vi "2022 Set Arm PID Constants.vi"(1 "error in (no error)":errorcluster, 2 "localConstantSpreadSheet":string[][](array[string]), 3 "robotID":string) -> (0 "error out":errorcluster)   [LabVIEW 2020]
uses:
  2023 Robot Global Data.vi
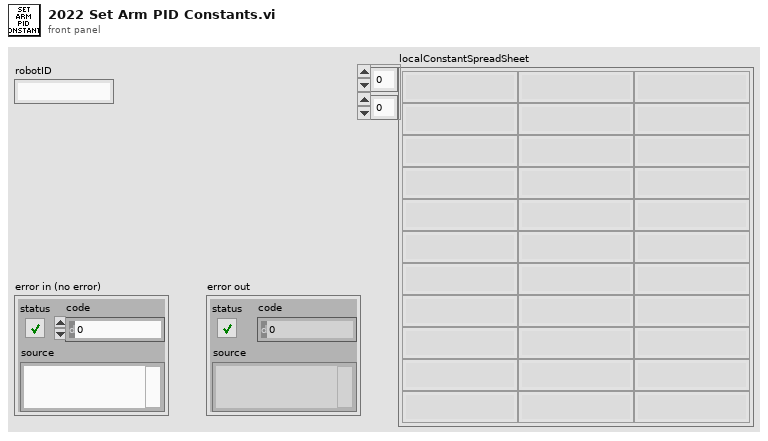
[diagram p1: front panel]
types:
  T1 = cluster{"P Gain":dbl, "I Gain":dbl, "D Gain":dbl, "F Gain":dbl, "I Zone":dbl, "Min Output":dbl, "Max Output":dbl}
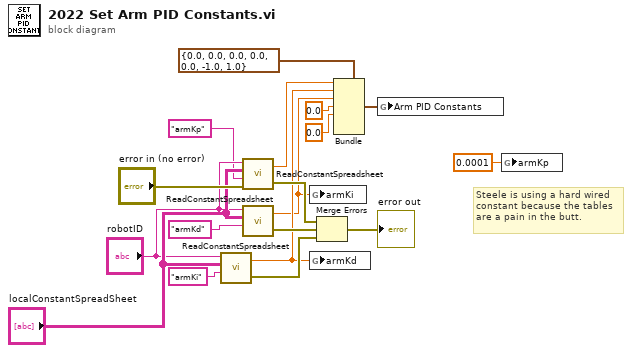
[diagram p0: block diagram]
diagram:
  # "Steele is using a hard wired\nconstant because the tables\nare a pain in the butt."
  n1 = call "ReadConstantSpreadsheet.vi"("Constant"="armKi", "2023ConstantSpreadSheet"="localConstantSpreadSheet", "Robot ID"="robotID") -> ("error out"=w16:errorcluster, "Constant Value"=w13:dbl)  [unwired: 1 in]
  n2 = call "ReadConstantSpreadsheet.vi"("error in"="error in (no error)", "Constant"="armKp", "2023ConstantSpreadSheet"="localConstantSpreadSheet", "Robot ID"="robotID") -> ("error out"=w14:errorcluster, "Constant Value"=w2:dbl)
  n3 = call "ReadConstantSpreadsheet.vi"("Constant"="armKd", "2023ConstantSpreadSheet"="localConstantSpreadSheet", "Robot ID"="robotID") -> ("error out"=w15:errorcluster, "Constant Value"=w12:dbl)  [unwired: 1 in]
  n4 = global write "2023 Robot Global Data.vi" "armKi"(w12) -> ()
  n5 = global write "2023 Robot Global Data.vi" "armKd"(w13) -> ()
  n6 = Merge Errors(w14, w15, w16) -> (→"error out":errorcluster)
  n7 = Bundle(cluster=T1 {"P Gain"=0.0, "I Gain"=0.0, "D Gain"=0.0, "F Gain"=0.0, "I Zone"=0.0, "Min Output"=-1.0, "Max Output"=1.0} ("PID Constants"), "P Gain"=w2, "I Gain"=w13, "D Gain"=w12, "F Gain"=0.0, "I Zone"=0.0) -> (w9:T1)  [unwired: 2 in]
  n8 = global write "2023 Robot Global Data.vi" "Arm PID Constants"(w9) -> ()
  n9 = global write "2023 Robot Global Data.vi" "armKp"(0.0001 ("armKp")) -> ()
